vi "Error Query.vi"(8 "error in (no error)":errorcluster, 11 "VISA resource name":refnum<visa-resource-name>) -> (0 "error out":errorcluster, 1 "Error Message":string, 2 "Error Code":i32[](array[numeric]), 3 "VISA resource name out":refnum<visa-resource-name>)   [LabVIEW 2025, in "Keithley 2182.lvlib"]
doc: "Queries the instrument for any errors in the instrument's error queue. It will continue to read errors until all errors have been read from the instrument. Any errors will be returned in the <B>error out</B> control.\n\n<B>Note:</B>\nThis VI is called automatically by most driver VIs so it is not usually necessary to call this in an application."
uses:
  Keithley 2182.lvlib
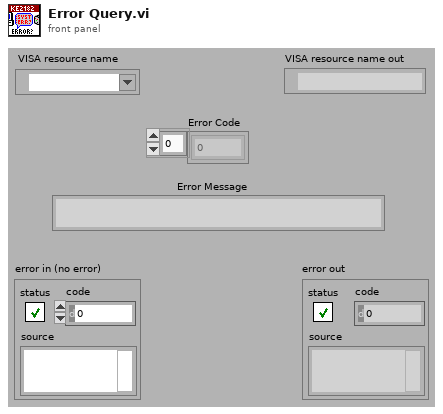
[diagram p1: front panel]
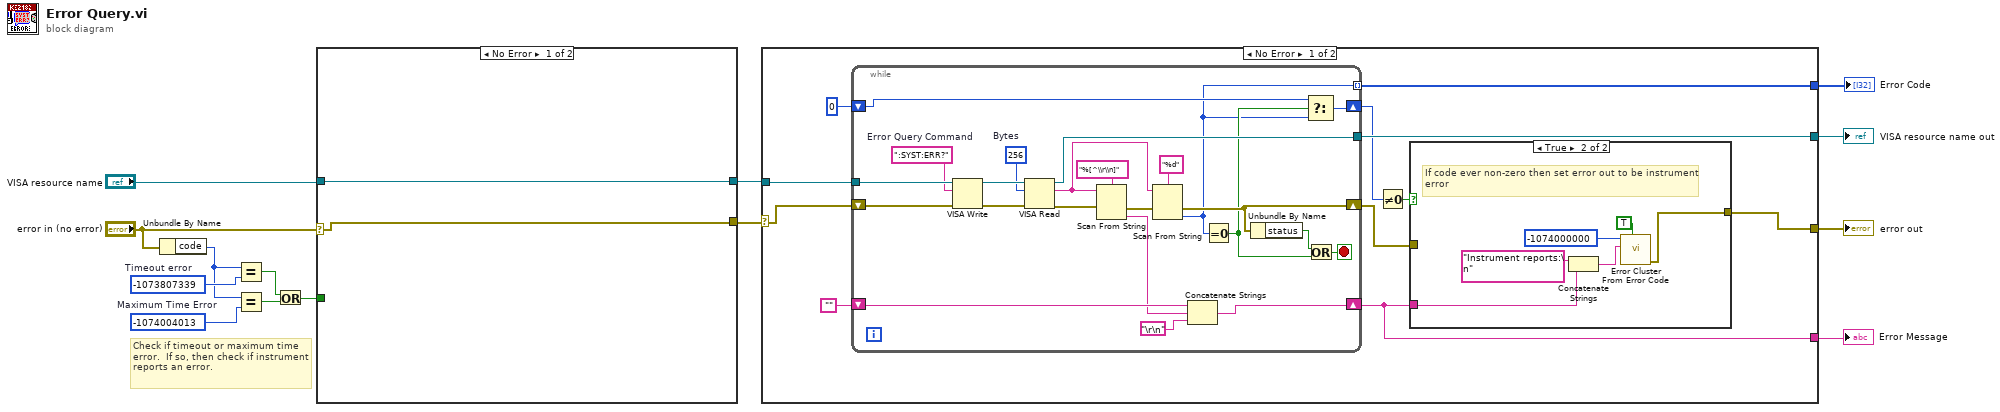
[diagram p0: block diagram]
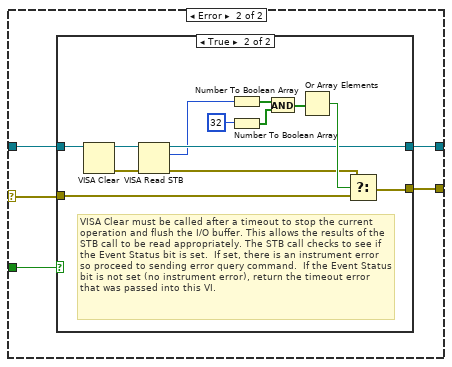
[diagram p2: hidden frame]
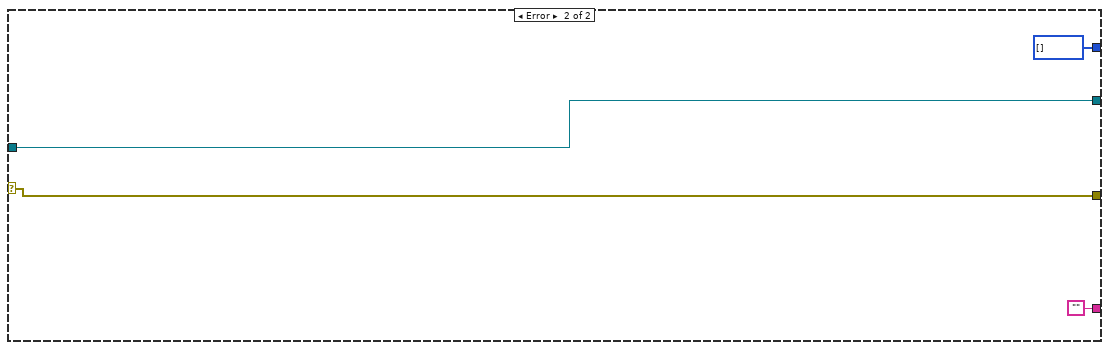
[diagram p5: hidden frame]
diagram:
  w5 = -1074004013  # Maximum Time Error
  w7 = -1073807339  # Timeout error
  # "Check if timeout or maximum time error.  If so, then check if instrument reports an error."
  n1 = Unbundle By Name("error in (no error)") -> ("code"=w6:i32)
  n2 = Equal?(x=w6, y=w7) -> (x = y?=w3:bool)
  n3 = Equal?(x=w6, y=w5) -> (x = y?=w4:bool)
  n4 = Or(x=w3, y=w4) -> (x .or. y?=w2:bool)
  n5 = case shown="No Error" "error in (no error)" {
    selector: "error in (no error)" -> [w15 w19]
    tunnel: "VISA resource name" -> [w16 w21]
    tunnel: [w16 w20] -> w9
    tunnel: [w15 w18] -> w10
    tunnel: w2 -> [_ w17]
    frame No Error {
    }
    frame Error {
      n6 = case shown="True" w17 {
        tunnel: w21 -> [w23 w29]
        tunnel: [w23 w26] -> w20
        tunnel: w19 -> [w22 w32]
        tunnel: [w22 w31] -> w18
        frame False {
          # "Error code not a timeout, so best to pass on to user."
        }
        frame True {
          # "VISA Clear must be called after a timeout to stop the current operation and flush the I/O buffer. This allows the results of the  STB call to be read appropriately. The STB call checks to see if the Event Status bit is set.  If set, there is an instrument error so proceed to sending error query command.  If the Event Status bit is not set (no instrument error), return the timeout error that was passed into this VI."
          n7 = VISA Clear(VISA resource name=w29) -> (VISA resource name out=w28:refnum<visa-resource-name>, error out=w27:errorcluster)  [unwired: 1 in]
          n8 = VISA Read STB(8:w27, 11:w28) -> (0:w25:errorcluster, 2:w24:u16, 3:w26:refnum<visa-resource-name>)
          n9 = Number To Boolean Array(number=w24) -> (Boolean array=w33:bool[])
          n10 = Number To Boolean Array(number=32) -> (Boolean array=w35:bool[])
          n11 = And(x=w33, y=w35) -> (x .and. y?=w34:bool[])
          n12 = Or Array Elements(Boolean array=w34) -> (logical OR=w30:bool)
          n13 = Select(t=w25, s=w30, f=w32) -> (s? t:f=w31:errorcluster)
        }
      }
    }
  }
  n14 = case shown="No Error" w10 {
    selector: w10 -> [w38 w78]
    tunnel: [w47 w81] -> w14
    tunnel: w9 -> [w46 w81]
    tunnel: [w37 w78] -> w13
    tunnel: [w41 ""] -> w12
    tunnel: [w40 i32[] []] -> w11
    frame No Error {
      n15 = while {
        tunnel: [w77] -> w47
        tunnel: w46 -> [w76]
        shift-right: [w64] -> w41
        shift-left: "" -> [w67]
        shift-right: [w62] -> w42
        shift-left: 0 -> [w63]
        shift-right: [w60] -> w39
        shift-left: w38 -> [w61]
        tunnel: [w55] -> w40 mode=indexing
        stop <- w70 stop-if-true
        w74 = u32 256  # Bytes
        w72 = ":SYST:ERR?"  # Error Query Command
        n16 = VISA Write(VISA resource name=w76, write buffer=w72, error in (no error)=w61) -> (VISA resource name out=w75:refnum<visa-resource-name>, error out=w73:errorcluster)  [unwired: 1 out]
        n17 = VISA Read(VISA resource name=w75, byte count=w74, error in (no error)=w73) -> (VISA resource name out=w77:refnum<visa-resource-name>, read buffer=w68:string, error out=w59:errorcluster)  [unwired: 1 out]
        n18 = Scan From String(format string="%[^\\r\\n]", input string=w68, error in=w59) -> (error out=w58:errorcluster, output 1=w65:string)  [unwired: 2 in, 2 out]
        n19 = Scan From String(format string="%d", input string=w68, error in=w58) -> (error out=w60:errorcluster, output 1=w55:i32)  [unwired: 2 in, 2 out]
        n20 = Concatenate Strings(w67, w65, "\r\n") -> (w64:string)
        n21 = Equal To 0?(x=w55) -> (x = 0?=w56:bool)
        n22 = Unbundle By Name(w60) -> ("status"=w57:bool)
        n23 = Select(t=w63, s=w56, f=w55) -> (s? t:f=w62:i32)
        n24 = Or(x=w57, y=w56) -> (x .or. y?=w70:bool)
      }
      n25 = Not Equal To 0?(x=w42) -> (x != 0?=w43:bool)
      n26 = case shown="True" w43 {
        tunnel: w41 -> [_ w53]
        tunnel: [w48 w49] -> w37
        tunnel: w39 -> [w48 _]
        frame False {
        }
        frame True {
          # "If code ever non-zero then set error out to be instrument error"
          n27 = Concatenate Strings("Instrument reports:\n" ("Source"), w53) -> (w50:string)
          n28 = call <vilib>:"Error Cluster From Error Code.vi"("show call chain? (False)"=TRUE, "error message (\"\")"=w50, "error code (0)"=-1074000000 ("Code")) -> ("error out"=w49:errorcluster)  [unwired: 6 in]
        }
      }
    }
    frame Error {
    }
  }
  "VISA resource name out" <- w14
  "error out" <- w13
  "Error Message" <- w12
  "Error Code" <- w11
